vi "servo_pickfromback_sequence.vi"(0 "servo 3":u8) -> ()   [LabVIEW 2017]
uses:
  GlobalVar.vi
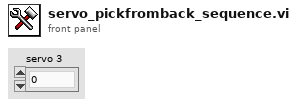
[diagram p1: front panel]
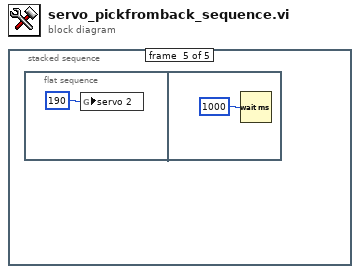
[diagram p0: block diagram]
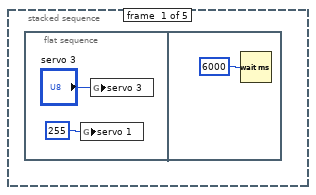
[diagram p2: hidden frame]
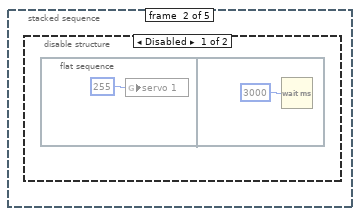
[diagram p3: hidden frame]
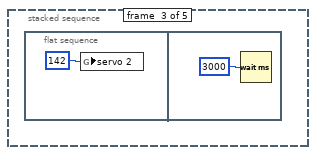
[diagram p5: hidden frame]
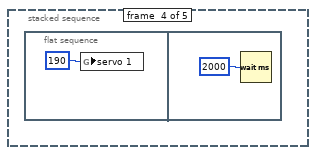
[diagram p6: hidden frame]
diagram:
  n1 = stacked-sequence {
    frame #0 {
      n2 = flat-sequence {
        frame #0 {
          n3 = global write "GlobalVar.vi" "servo 1"(u8 255 ("servo 1")) -> ()
          n4 = global write "GlobalVar.vi" "servo 3"("servo 3") -> ()
        }
        frame #1 {
          n5 = Wait (ms)(milliseconds to wait=u32 6000) -> ()  [unwired: 1 out]
        }
      }
    }
    frame #1 {
      n6 = disable-structure shown="Disabled" {
        frame Disabled {
          n7 = flat-sequence {
            frame #0 {
              n8 = global write "GlobalVar.vi" "servo 1"(u8 255 ("servo 1")) -> ()
            }
            frame #1 {
              n9 = Wait (ms)(milliseconds to wait=u32 3000) -> ()  [unwired: 1 out]
            }
          }
        }
        frame Enabled {
        }
      }
    }
    frame #2 {
      n10 = flat-sequence {
        frame #0 {
          n11 = global write "GlobalVar.vi" "servo 2"(u8 142 ("servo 1")) -> ()
        }
        frame #1 {
          n12 = Wait (ms)(milliseconds to wait=u32 3000) -> ()  [unwired: 1 out]
        }
      }
    }
    frame #3 {
      n13 = flat-sequence {
        frame #0 {
          n14 = global write "GlobalVar.vi" "servo 1"(u8 190 ("servo 1")) -> ()
        }
        frame #1 {
          n15 = Wait (ms)(milliseconds to wait=u32 2000) -> ()  [unwired: 1 out]
        }
      }
    }
    frame #4 {
      n16 = flat-sequence {
        frame #0 {
          n17 = global write "GlobalVar.vi" "servo 2"(u8 190 ("servo 1")) -> ()
        }
        frame #1 {
          n18 = Wait (ms)(milliseconds to wait=u32 1000) -> ()  [unwired: 1 out]
        }
      }
    }
  }
